vi "Import-RGB_to_HSV.vi"(8 "Error In (no error)":errorcluster, 11 "RGB":u8[](array[numeric])) -> (0 "Error Out":errorcluster, 1 "Value":dbl, 2 "Saturation":dbl, 3 "Hue in degrees":dbl)   [LabVIEW 2020]
doc: "<B>Description:</B> Converts 16 bit RGB values to Hue, Saturation and Value\n\n<B>Date:</B> 08/2018\n<B>Author:</B> Luke Jarocki, Choose Movement Consulting, LLC"
panel:
  out "Case":string
  out "Blue":u8
  out "Green":u8
  out "Red":u8
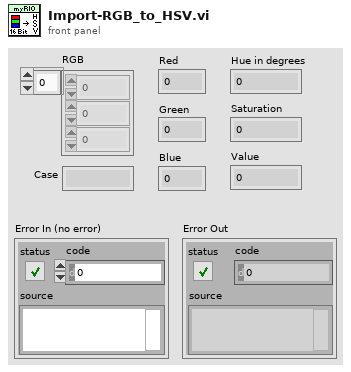
[diagram p1: front panel]
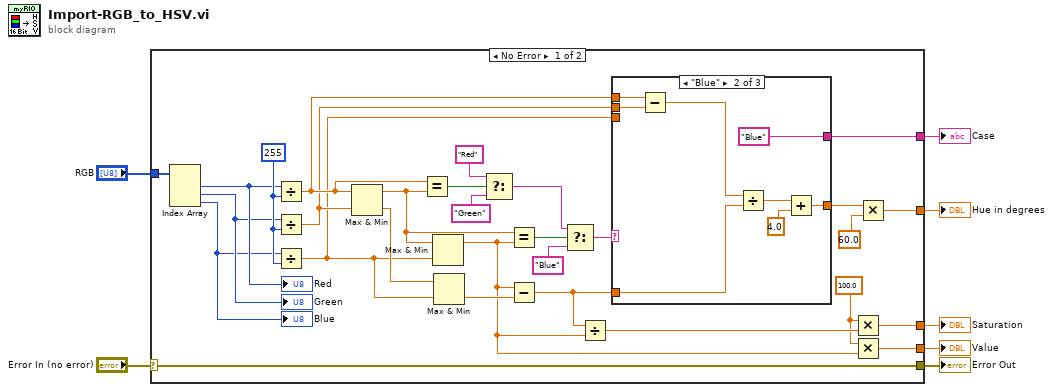
[diagram p0: block diagram]
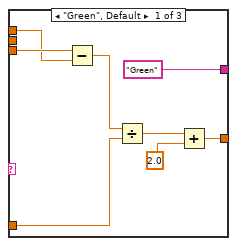
[diagram p2: hidden frame]
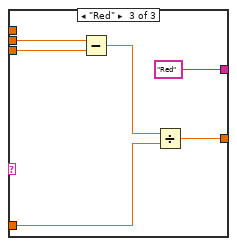
[diagram p3: hidden frame]
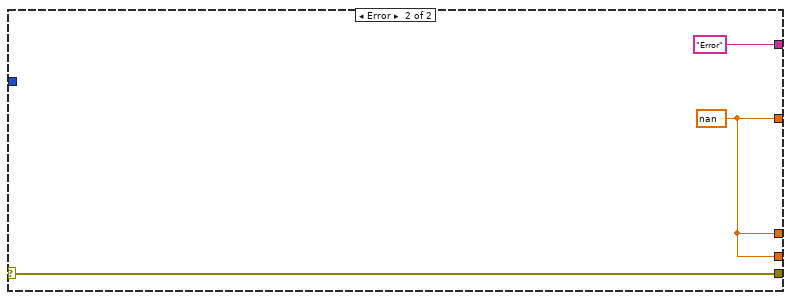
[diagram p4: hidden frame]
diagram:
  n1 = case shown="No Error" "Error In (no error)" {
    selector: "Error In (no error)" -> [w13 w60]
    tunnel: [w25 "Error"] -> w7
    tunnel: [w11 w59] -> w6
    tunnel: [w22 w59] -> w5
    tunnel: "RGB" -> [w17 _]
    tunnel: [w13 w60] -> w2
    tunnel: [w8 w59] -> w1
    frame No Error {
      w9 = 100.0 ("x")
      w24 = u16 255 ("y")
      n2 = Index Array(array=w17) -> (element #1=w16:u8, element #2=w15:u8, element #3=w14:u8)  [unwired: 3 in]
      "Red" <- w16
      "Green" <- w15
      "Blue" <- w14
      n3 = Divide(x=w16, y=w24) -> (x/y=w21:dbl)
      n4 = Divide(x=w15, y=w24) -> (x/y=w20:dbl)
      n5 = Divide(x=w14, y=w24) -> (x/y=w19:dbl)
      n6 = Max & Min(x=w21, y=w20) -> (max(x,y)=w33:dbl, min(x,y)=w28:dbl)
      n7 = Equal?(x=w21, y=w33) -> (x = y?=w36:bool)
      n8 = Max & Min(x=w33, y=w19) -> (max(x,y)=w10:dbl)  [unwired: 1 out]
      n9 = Max & Min(x=w28, y=w19) -> (min(x,y)=w18:dbl)  [unwired: 1 out]
      n10 = Select(t="Red", s=w36, f="Green") -> (s? t:f=w32:string)
      n11 = Equal?(x=w33, y=w10) -> (x = y?=w30:bool)
      n12 = Subtract(x=w10, y=w18) -> (x-y=w23:dbl)
      n13 = Select(t=w32, s=w30, f="Blue") -> (s? t:f=w29:string)
      n14 = Divide(x=w23, y=w10) -> (x/y=w12:dbl)
      n15 = case shown="\"Blue\"" w29 {
        tunnel: w23 -> [w40 w48 w55]
        tunnel: w21 -> [w42 w47 _]
        tunnel: w20 -> [_ w46 w58]
        tunnel: w19 -> [w43 _ w57]
        tunnel: [w37 w45 w54] -> w27
        tunnel: ["Green" "Blue" "Red"] -> w25
        frame "Green", Default {
          n16 = Subtract(x=w43, y=w42) -> (x-y=w41:dbl)
          n17 = Divide(x=w41, y=w40) -> (x/y=w39:dbl)
          n18 = Add(x=w39, y=2.0) -> (x+y=w37:dbl)
        }
        frame "Blue" {
          n19 = Subtract(x=w47, y=w46) -> (x-y=w51:dbl)
          n20 = Divide(x=w51, y=w48) -> (x/y=w50:dbl)
          n21 = Add(x=w50, y=4.0) -> (x+y=w45:dbl)
        }
        frame "Red" {
          n22 = Subtract(x=w58, y=w57) -> (x-y=w56:dbl)
          n23 = Divide(x=w56, y=w55) -> (x/y=w54:dbl)
        }
      }
      n24 = Multiply(x=w9, y=w12) -> (x*y=w11:dbl)
      n25 = Multiply(x=w9, y=w10) -> (x*y=w8:dbl)
      n26 = Multiply(x=w27, y=60.0) -> (x*y=w22:dbl)
    }
    frame Error {
      w59 = nan
    }
  }
  "Hue in degrees" <- w5
  "Case" <- w7
  "Saturation" <- w6
  "Error Out" <- w2
  "Value" <- w1
